vi "Exemple_Preprocessing_OneHotEncoder.vi"() -> ()   [LabVIEW 2020]
uses:
  Objet/6 - Datasets Transformation/6.3 - Processing Data/OneHotEncoder/OneHotEncoder.lvclass
panel:
  in  "y":string[][](array[string])
  in  "X":string[][](array[string])=[["Male", "1"], ["Female", "3"], ["Female", "2"]]
  out "Data":T1
  out "error out":errorcluster
  in  "error in":errorcluster caption="entrée d'erreur"
  in  "OneHotEncoder":T2={"drop"="None", "sparse"=TRUE, "dtype"="float", "handle_unknown"="error"}
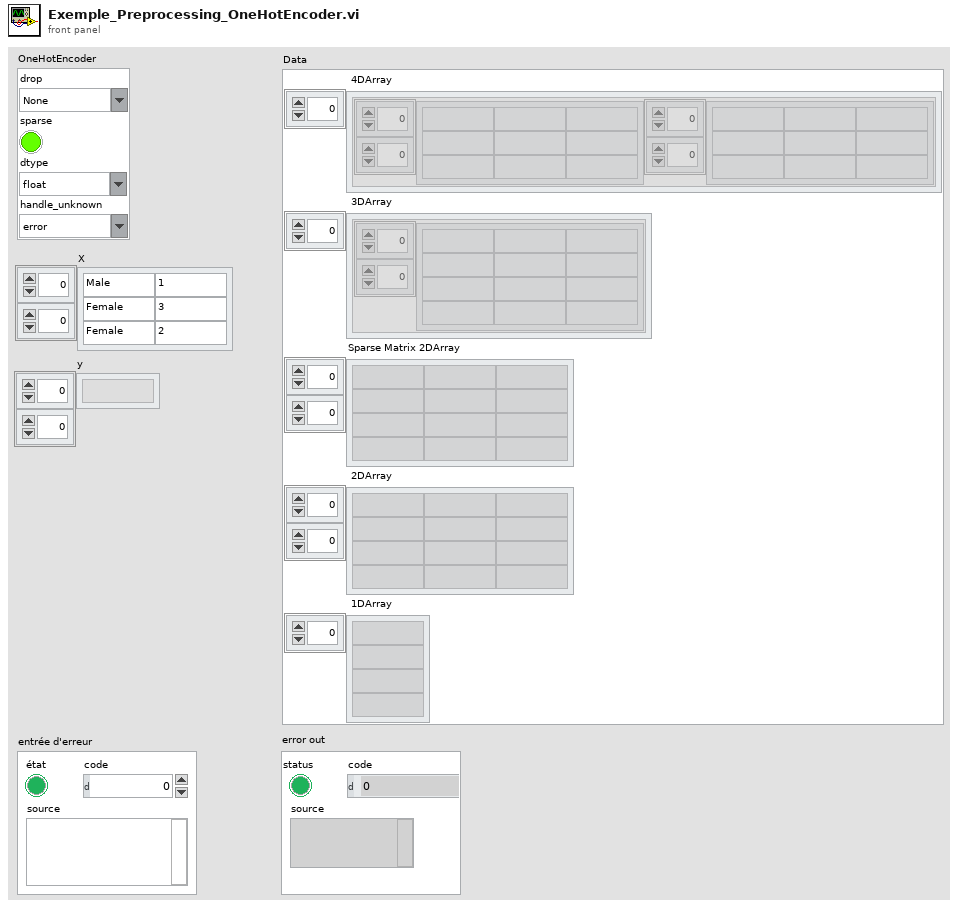
[diagram p1: front panel]
types:
  T1 = cluster{" 4DArray":cluster{"1":string[][], "2":string[][]}[], " 3DArray":cluster{"Tableau":string[][]}[], "Sparse Matrix 2DArray":string[][], " 2DArray":string[][], " 1DArray":string[]}
  T2 = cluster{"drop":string, "sparse":bool, "dtype":string, "handle_unknown":string}
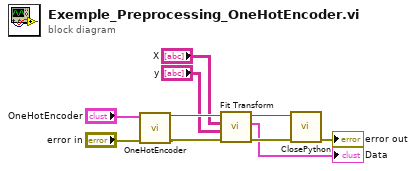
[diagram p0: block diagram]
diagram:
  n1 = call "OneHotEncoder.vi"("error in (no error)"="error in", "OneHotEncoder"="OneHotEncoder") -> ("error out"=w8:errorcluster, "OneHotEncoder.lvclass"=w7:refnum<class "OneHotEncoder.lvclass">)  [unwired: 8 in]
  n2 = call-dynamic "Fit Transform.vi"("error in (no error)"=w8, "y"="y", "X"="X", "OneHotEncoder.lvclass"=w7) -> ("error out"=w5:errorcluster, "Data"=→"Data":T1, "OneHotEncoder.lvclass"=w6:refnum<class "OneHotEncoder.lvclass">)  [unwired: 5 in]
  n3 = call-dynamic "ClosePython.vi"("error in (no error)"=w5, "Scikit-learn en entrée"=w6) -> ("error out"=→"error out":errorcluster)  [unwired: 8 in, 1 out]
